vi "Initialize.vi"(8 "error in (no error)":errorcluster, 10 "Config":T1[](array[typedef]), 11 "Device in":refnum<class "Device.lvclass">) -> (0 "error out":errorcluster, 3 "Device out":refnum<class "Device.lvclass">)   [LabVIEW 2020, in "HAL.lvlib" / "Device.lvclass"]
uses:
  Device.lvclass
  Config Item.ctl
  Ref Data.ctl
  Device State.ctl
  Device.lvclass/Device.ctl
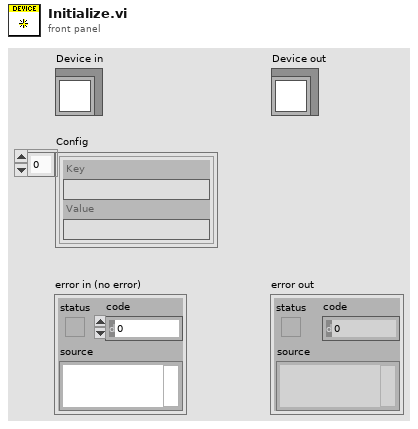
[diagram p1: front panel]
types:
  T1 = typedef "HAL.lvlib/Device.lvclass/Config Item.ctl" = cluster{"Key":string, "Value":string}
  T2 = typedef "HAL.lvlib/Device.lvclass/Device State.ctl" = enum16{"Uninitialized", "Initialized", "Running", "Error"}
  T3 = typedef "HAL.lvlib/Device.lvclass/Ref Data.ctl" = cluster{"Config Keys":string[], "Config Values":string[], "Cal Expires":timestamp, "Name":string, "Comment":string, "State":T2, "Error":errorcluster}
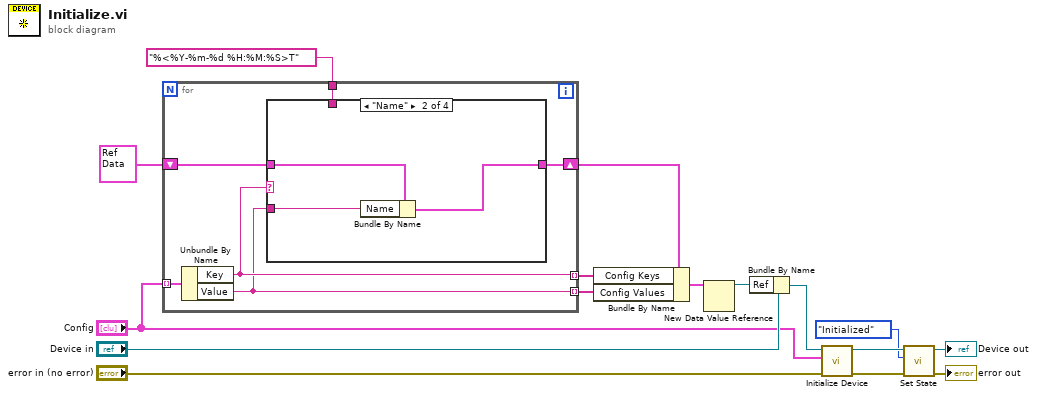
[diagram p0: block diagram]
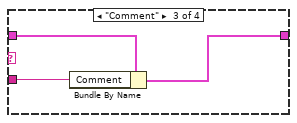
[diagram p3: hidden frame]
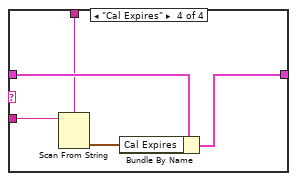
[diagram p4: hidden frame]
diagram:
  n1 = for {
    shift-right: [w18] -> w11
    shift-left: T3 {"Config Keys"=[], "Config Values"=[], "Cal Expires"=timestamp(0 s since 1904-01-01), "Name"="", "Comment"="", "State"=enum."Uninitialized", "Error"={"status"=FALSE, "code"=0, "source"=""}} ("Ref Data") -> [w19]
    tunnel: "Config" -> [w22] mode=indexing
    tunnel: [w20] -> w9 mode=indexing
    tunnel: [w21] -> w10 mode=indexing
    tunnel: "%<%Y-%m-%d %H:%M:%S>T" ("format string") -> [w17]
    n2 = Unbundle By Name(w22) -> ("Key"=w21:string, "Value"=w20:string)
    n3 = case shown="\"Name\"" w21 {
      tunnel: w20 -> [_ w25 w28 w32]
      tunnel: w19 -> [w23 w26 w29 w34]
      tunnel: [w23 w24 w27 w33] -> w18
      tunnel: w17 -> [_ _ _ w31]
      frame Default {
      }
      frame "Name" {
        n4 = Bundle By Name(cluster=w26, "Name"=w25) -> (w24:T3)
      }
      frame "Comment" {
        n5 = Bundle By Name(cluster=w29, "Comment"=w28) -> (w27:T3)
      }
      frame "Cal Expires" {
        n6 = Scan From String(format string=w31, input string=w32) -> (output 1=w30:timestamp)  [unwired: 3 in, 3 out]
        n7 = Bundle By Name(cluster=w34, "Cal Expires"=w30) -> (w33:T3)
      }
    }
  }
  n8 = Bundle By Name(cluster=w11, "Config Keys"=w10, "Config Values"=w9) -> (w8:T3)
  n9 = New Data Value Reference(data value=w8) -> (data value reference=w7:refnum<data-value>)  [unwired: 1 in, 1 out]
  n10 = Bundle By Name(cluster="Device in", "Ref"=w7) -> (w14:refnum<class "Device.lvclass">)
  n11 = call-dynamic "Initialize Device.vi"("error in (no error)"="error in (no error)", "Config"="Config", "Device in"=w14) -> ("error out"=w4:errorcluster, "Device out"=w5:refnum<class "Device.lvclass">)  [unwired: 7 in]
  n12 = call "Set State.vi"("error in (no error)"=w4, "Device State"=Device_State."Initialized", "Device in"=w5) -> ("error out"=→"error out":errorcluster, "Device out"=→"Device out":refnum<class "Device.lvclass">)  [unwired: 7 in]
